vi "GuiLogIn.vi"() -> ()   [LabVIEW 2019]
panel:
  in  "jr 2":bool
  in  "jr":bool
  in  "pass":string
  in  "login":string
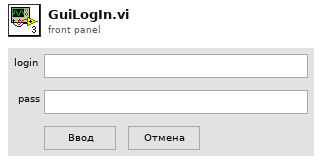
[diagram p1: front panel]
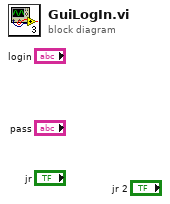
[diagram p0: block diagram]
diagram:
